vi "fake resource long string.vi"(11 "input string":string) -> (3 "resulting string":string)   [LabVIEW 2025, in "MCP Server tests.lvlib"]
doc: "A resource that returns a long string containing an input string."
uses:
  MCP Server tests.lvlib
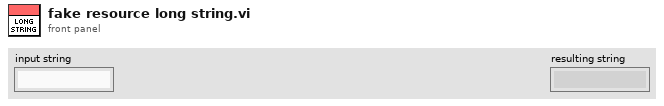
[diagram p1: front panel]
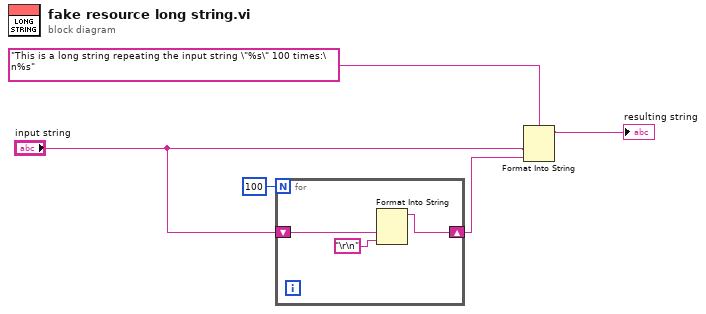
[diagram p0: block diagram]
diagram:
  n1 = for {
    N: 100 -> [_]
    shift-right: [w6] -> w3
    shift-left: "input string" -> [w8]
    n2 = Format Into String(w8, "\r\n") -> (resulting string=w6:string)  [unwired: 3 in, 1 out]
  }
  n3 = Format Into String(format string="This is a long string repeating the input string \"%s\" 100 times:\n%s", "input string", w3) -> (resulting string=→"resulting string":string)  [unwired: 2 in, 1 out]
